vi "Yuval Algo extracted.vi"() -> ()   [LabVIEW 2015]
uses:
  algo1.vi
panel:
  in  "stop":bool
  out "Time":u32
  out "Number of Matches (Shape Detection 1)":i32
  in  "Range (Threshold 1)":cluster{"Lower value":sgl, "Upper value":sgl}={"Lower value"=0.0, "Upper value"=195.0}
  out "Circles Calibrated (Shape Detection 1)":T1(array[cluster]) {"Position"."Y" format="%.2f"; "Position"."X" format="%.2f"}
  out "Circles (Shape Detection 1)":T1(array[cluster]) {"Position"."Y" format="%.2f"; "Position"."X" format="%.2f"}
  out "error out 2":errorcluster
  out "error out":errorcluster
  out "Image Out":T2(plugin-control)
  out "Image In":T2(plugin-control)
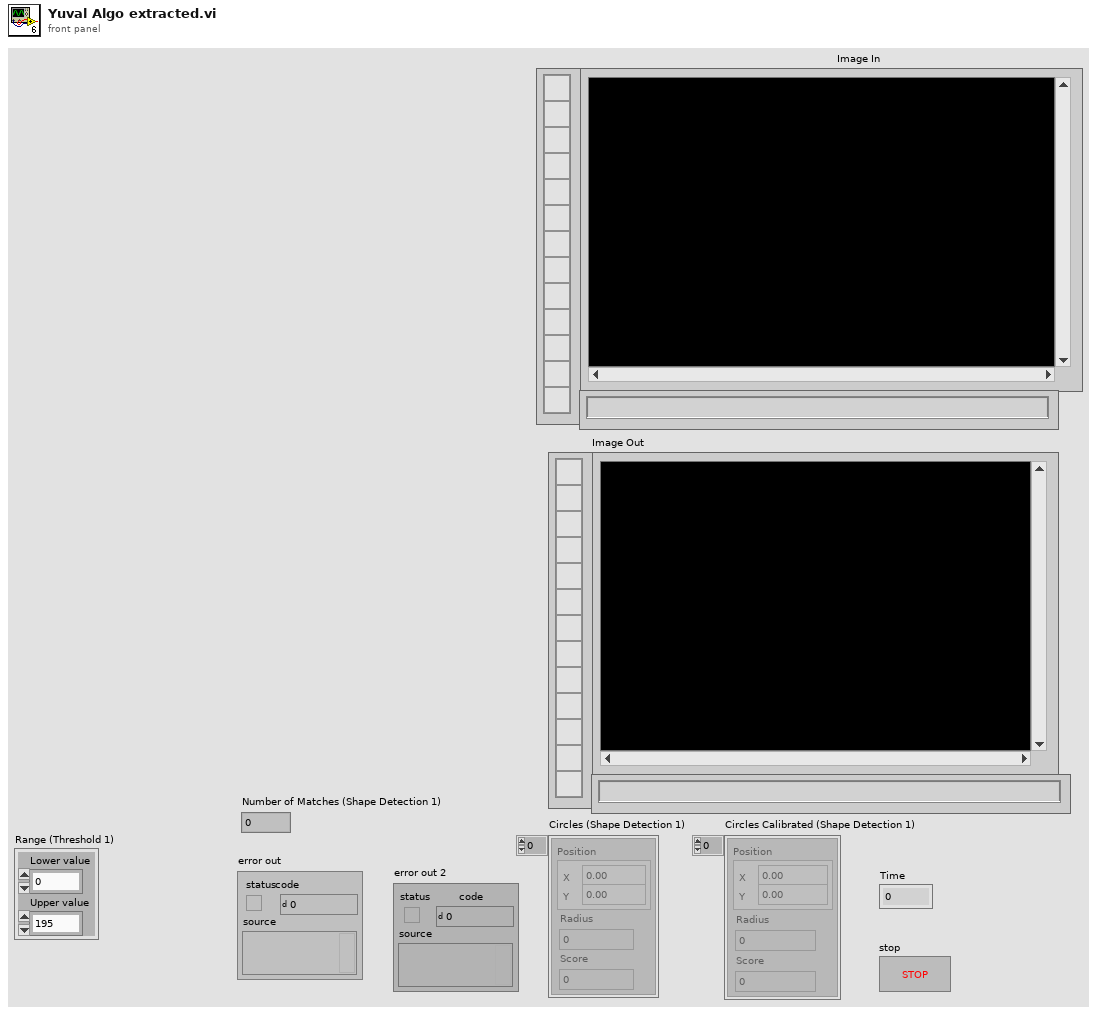
[diagram p1: front panel]
types:
  T1 = cluster{"Position":cluster{"X":sgl, "Y":sgl}, "Radius":dbl, "Score":dbl}[]
  T2 = typedef "IMAQ Image.ctl" = refnum<image>
  T3 = cluster{"Rotation":bool, "Scale":bool, "Occlusion":bool, "Range Settings":cluster{"Match Constraints":u32, "Min":dbl, "Max":dbl}[]}
  T4 = typedef "Image Type" = u32
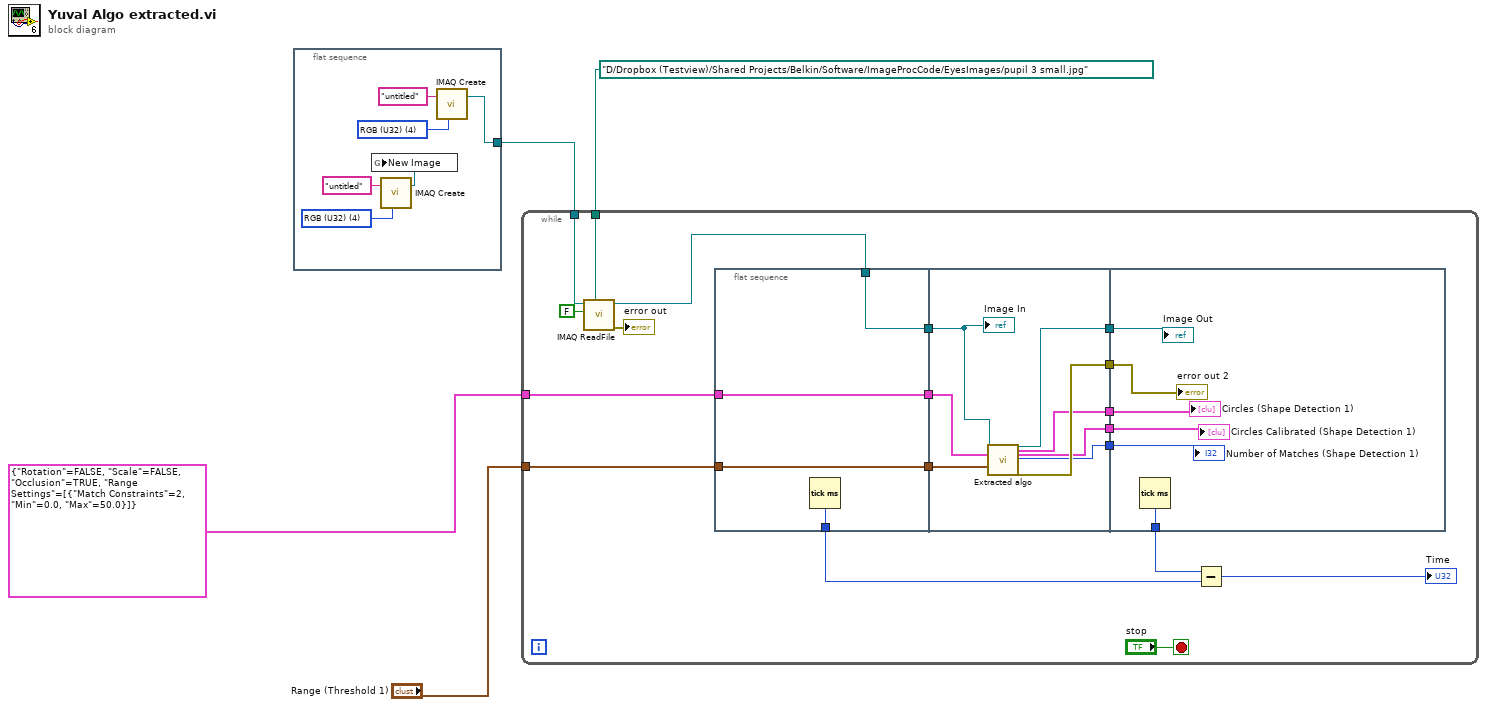
[diagram p0: block diagram]
diagram:
  n1 = flat-sequence {
    tunnel: [w8] -> w1
    frame #0 {
      w7 = T4 4 items=["Grayscale (U8)", "Grayscale (I16)", "Grayscale (SGL)", "Complex (CSG)", "RGB (U32)", "HSL (U32)", "RGB (U64)", "Grayscale (U16)"] ("Image Type")
      w10 = T4 4 items=["Grayscale (U8)", "Grayscale (I16)", "Grayscale (SGL)", "Complex (CSG)", "RGB (U32)", "HSL (U32)", "RGB (U64)", "Grayscale (U16)"] ("Image Type")
      n2 = call "IMAQ Create"("Image Name"="untitled", "Image Type"=w7) -> ("New Image"=w5:T2)  [unwired: 2 in, 2 out]
      n3 = global write "algo1.vi" "New Image"(w5) -> ()
      n4 = call "IMAQ Create"("Image Name"="untitled", "Image Type"=w10) -> ("New Image"=w8:T2)  [unwired: 2 in, 2 out]
    }
  }
  n5 = while {
    tunnel: T3 {"Rotation"=FALSE, "Scale"=FALSE, "Occlusion"=TRUE, "Range Settings"=[{"Match Constraints"=2, "Min"=0.0, "Max"=50.0}]} ("Match Options (Shape Detection 1)") -> [w29]
    tunnel: "Range (Threshold 1)" -> [w28]
    tunnel: path "D:/Dropbox (Testview)/Shared Projects/Belkin/Software/ImageProcCode/EyesImages/pupil 3 small.jpg" ("File Path") -> [w13]
    tunnel: w1 -> [w12]
    stop <- "stop" stop-if-true
    n6 = call "IMAQ ReadFile"("File Path"=w13, "Load Color Palette? (No)"=FALSE, "Image"=w12) -> ("error out"=→"error out":errorcluster, "Image Out"=w11:T2)  [unwired: 4 in, 3 out]
    n7 = flat-sequence {
      tunnel: w28 -> [w32]
      tunnel: w29 -> [w33]
      tunnel: [w33] -> w27
      tunnel: [w32] -> w26
      tunnel: [w31] -> w20
      tunnel: [w30] -> w17
      tunnel: w11 -> [w30]
      tunnel: w27 -> [w40]
      tunnel: w26 -> [w37]
      tunnel: [w41] -> w25
      tunnel: [w39] -> w24
      tunnel: [w38] -> w23
      tunnel: [w36] -> w22
      tunnel: w17 -> [w34]
      tunnel: [w35] -> w16
      tunnel: w25 -> [w46]
      tunnel: w24 -> [w44]
      tunnel: w23 -> [w43]
      tunnel: w22 -> [w42]
      tunnel: [w47] -> w21
      tunnel: w16 -> [w45]
      frame #0 {
        n8 = Tick Count (ms)() -> (millisecond timer value=w31:u32)
      }
      frame #1 {
        n9 = call "Extracted algo.vi"("Image In"=w34, "Match Options (Shape Detection 1)"=w40, "Range (Threshold 1)"=w37) -> ("Image Out"=w35:T2, "Circles (Shape Detection 1)"=w39:T1, "Circles Calibrated (Shape Detection 1)"=w38:T1, "Number of Matches (Shape Detection 1)"=w36:i32, "error out"=w41:errorcluster)  [unwired: 20 in]
        "Image In" <- w34
      }
      frame #2 {
        n10 = Tick Count (ms)() -> (millisecond timer value=w47:u32)
        "error out 2" <- w46
        "Circles (Shape Detection 1)" <- w44
        "Circles Calibrated (Shape Detection 1)" <- w43
        "Number of Matches (Shape Detection 1)" <- w42
        "Image Out" <- w45
      }
    }
    n11 = Subtract(x=w21, y=w20) -> (x-y=→"Time":u32)
  }
